vi "2 Round Buoy.vi"() -> ()   [LabVIEW 2011]
uses:
  2 Globals/2 Global.vi
  2 Typedefs/Velocity.ctl
  2 Typedefs/UTM Location.ctl
  2 Classes/Mission/Mission.lvclass
  2 Classes/MissionQueue/MissionQueue.lvclass
  2 Classes/Waypoint/Waypoint.lvclass
panel:
  in  "Tolerance":dbl=0.5
  out "First Waypoint":T1 {"North" format="%#_10f"; "East" format="%#_8f"}
  out "Third Waypoint":T1 {"North" format="%#_10f"; "East" format="%#_8f"}
  out "Second Waypoint":T1 {"North" format="%#_10f"; "East" format="%#_8f"}
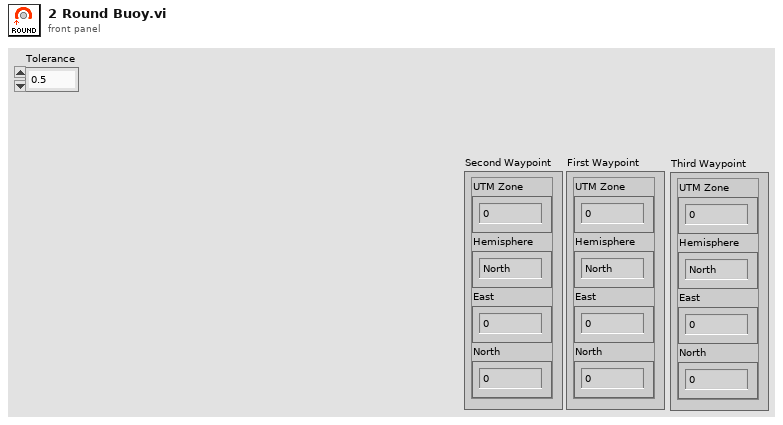
[diagram p1: front panel]
types:
  T1 = typedef "UTM Location.ctl" = cluster{"UTM Zone":dbl, "Hemisphere":enum16{"North", "South"}, "East":dbl, "North":dbl}
  T2 = typedef "Velocity.ctl" = cluster{"East":dbl, "North":dbl}
  T3 = cluster{"UTM Zone":dbl, "Hemisphere":u16, "East":dbl, "North":dbl}
  T4 = typedef "heading.ctl" = dbl
  T5 = typedef "Waypoints List.ctl" = refnum<class "Waypoint.lvclass">[]
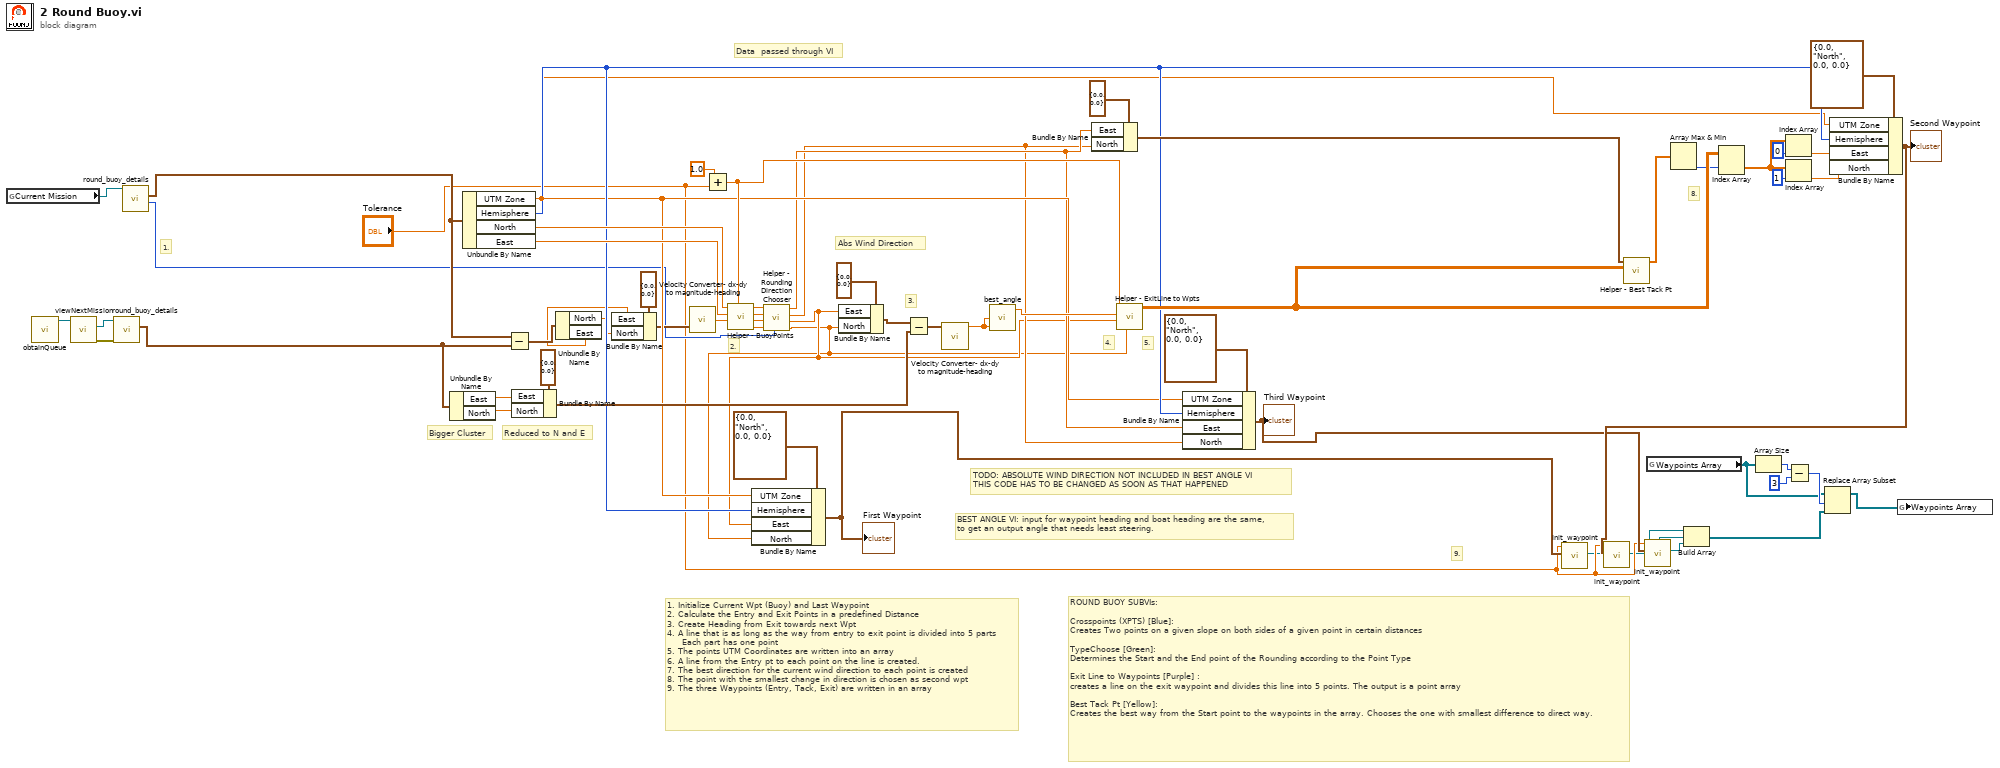
[diagram p0: block diagram]
diagram:
  # "ROUND BUOY SUBVIs:\n\nCrosspoints (XPTS) [Blue]:\nCreates Two points on a given slope on both sides of a given point in certain distances\n\nTypeChoose [Green]:\nDetermines the Start and the End point of the Rounding according to the Point Type\n\nExit Line to Waypoints [Purple] :\ncreates a line on the exit waypoint and divides this line into 5 points. The output is a point array\n\nBest Tack Pt [Yellow]:\nCreates the best way from the Start point to the waypoints in the array. Chooses the one with smallest difference to direct way."
  # "BEST ANGLE VI: input for waypoint heading and boat heading are the same,\nto get an output angle that needs least steering."
  # "Reduced to N and E"
  # "Bigger Cluster"
  # "Data  passed through VI"
  # "9."
  # "TODO: ABSOLUTE WIND DIRECTION NOT INCLUDED IN BEST ANGLE VI\nTHIS CODE HAS TO BE CHANGED AS SOON AS THAT HAPPENED"
  # "8."
  # "5."
  # "1. Initialize Current Wpt (Buoy) and Last Waypoint\n2. Calculate the Entry and Exit Points in a predefined Distance\n3. Create Heading from Exit towards next Wpt\n4. A line that is as long as the way from entry to exit point is divided into 5 parts\n     Each part has one point\n5. The points UTM Coordinates are written into an array\n6. A line from the Entry pt to each point on the line is created.\n7. The best direction for the current wind direction to each point is created\n8. The point with the smallest change in direction is chosen as second wpt\n9. The three Waypoints (Entry, Tack, Exit) are written in an array"
  # "4."
  # "3."
  # "Abs Wind Direction"
  # "2."
  # "1."
  n1 = global read "2 Global.vi" "Current Mission"() -> (w21:refnum<class "Mission.lvclass">)
  n2 = call "obtainQueue.vi"() -> ("MissionQueue.lvclass"=w15:refnum<class "MissionQueue.lvclass">)  [unwired: 10 in, 1 out]
  n3 = call "viewNextMission.vi"("MissionQueue in"=w15) -> ("error out"=w18:errorcluster, "Mission.lvclass"=w17:refnum<class "Mission.lvclass">)  [unwired: 7 in, 2 out]
  n4 = call-dynamic "round_buoy_details.vi"("error in (no error)"=w18, "Mission in"=w17) -> ("Buoy to Round"=w16:T1)  [unwired: 6 in, 3 out]
  n5 = call-dynamic "round_buoy_details.vi"("Mission in"=w21) -> ("Round side?"=w19:enum16{"Starboard", "Port"}, "Buoy to Round"=w20:T1)  [unwired: 7 in, 2 out]
  n6 = Unbundle By Name(w16) -> ("East"=w59:dbl, "North"=w58:dbl)
  n7 = Unbundle By Name(w20) -> ("UTM Zone"=w36:dbl, "Hemisphere"=w37:enum16{"North", "South"}, "North"=w62:dbl, "East"=w61:dbl)
  n8 = Subtract(x=w20, y=w16) -> (x-y=w26:T3)
  n9 = Bundle By Name(cluster=T2 {"East"=0.0, "North"=0.0} ("Vector In"), "East"=w59, "North"=w58) -> (w55:T2)
  n10 = Unbundle By Name(w26) -> ("North"=w24:dbl, "East"=w14:dbl)
  n11 = Bundle By Name(cluster=T2 {"East"=0.0, "North"=0.0} ("Vector In"), "East"=w14, "North"=w24) -> (w23:T2)
  n12 = call "Velocity Converter- dx-dy to magnitude-heading.vi"("Vector In"=w23) -> ("Heading Out"=w22:T4)  [unwired: 9 in, 1 out]
  n13 = Add(x=1.0, y="Tolerance") -> (x+y=w53:dbl)
  n14 = call "Helper - BuoyPoints.vi"("Distance"=w53, "K"=w22, "East"=w61, "North"=w62) -> ("NorthOut 2"=w31:dbl, "East Out 2"=w32:dbl, "NorthOut"=w33:dbl, "East Out"=w34:dbl)  [unwired: 4 in]
  n15 = call "Helper - Rounding Direction Chooser.vi"("Enum"=w19, "Point NORTH 2"=w31, "Point EAST 2"=w32, "Point NORTH"=w33, "Point EAST"=w34) -> ("End Point NORTH"=w27:dbl, "End Point EAST"=w28:dbl, "Start Point NORTH"=w29:dbl, "Start Point EAST"=w30:dbl)  [unwired: 3 in]
  n16 = Bundle By Name(cluster=T1 {"UTM Zone"=0.0, "Hemisphere"=enum."North", "East"=0.0, "North"=0.0} ("UTM Location"), "UTM Zone"=w36, "Hemisphere"=w37, "East"=w28, "North"=w27) -> (w13:T1)
  "First Waypoint" <- w13
  n17 = Bundle By Name(cluster=T2 {"East"=0.0, "North"=0.0} ("Vector In"), "East"=w28, "North"=w27) -> (w41:T2)
  n18 = Subtract(x=w41, y=w55) -> (x-y=w54:T2)
  n19 = call "Velocity Converter- dx-dy to magnitude-heading.vi"("Vector In"=w54) -> ("Heading Out"=w35:T4)  [unwired: 9 in, 1 out]
  n20 = call "best_angle.vi"("Waypoint Heading"=w35, "Current Heading"=w35) -> ("Best Angle"=w52:dbl)  [unwired: 1 in, 2 out]
  n21 = Bundle By Name(cluster=T2 {"East"=0.0, "North"=0.0} ("Vector In"), "East"=w30, "North"=w29) -> (w42:T2)
  n22 = call "Helper - ExitLine to Wpts.vi"("NorthOut in"=w27, "East Out in"=w28, "Best Angle"=w52, "Dist/Time"=w53) -> ("Point on Line"=w49:dbl[][])  [unwired: 7 in]
  n23 = Bundle By Name(cluster=T1 {"UTM Zone"=0.0, "Hemisphere"=enum."North", "East"=0.0, "North"=0.0} ("UTM Location"), "UTM Zone"=w36, "Hemisphere"=w37, "East"=w30, "North"=w29) -> (w11:T1)
  "Third Waypoint" <- w11
  n24 = call "init_waypoint.vi"("Coords"=w13, "Tolerance (m)"="Tolerance") -> ("Waypoint Out"=w8:refnum<class "Waypoint.lvclass">)  [unwired: 9 in]
  n25 = call "Helper - Best Tack Pt.vi"("Point on Line"=w49, "Vector In"=w42) -> ("Array"=w50:dbl[])  [unwired: 9 in]
  n26 = call "init_waypoint.vi"("Coords"=w11, "Tolerance (m)"="Tolerance") -> ("Waypoint Out"=w6:refnum<class "Waypoint.lvclass">)  [unwired: 9 in]
  n27 = global read "2 Global.vi" "Waypoints Array"() -> (w3:T5)
  n28 = Array Max & Min(array=w50) -> (min index (indices)=w48:i32)  [unwired: 3 out]
  n29 = Index Array(array=w49, index (row)=w48) -> (element=w43:dbl[])  [unwired: 1 in]
  n30 = Array Size(array=w3) -> (size(s)=w9:i32)
  n31 = Index Array(array=w43, index=0) -> (element=w45:dbl)
  n32 = Index Array(array=w43, index=1) -> (element=w44:dbl)
  n33 = Subtract(x=w9, y=3) -> (x-y=w4:i32)
  n34 = Bundle By Name(cluster=T1 {"UTM Zone"=0.0, "Hemisphere"=enum."North", "East"=0.0, "North"=0.0} ("UTM Location"), "UTM Zone"=w36, "Hemisphere"=w37, "East"=w45, "North"=w44) -> (w12:T1)
  "Second Waypoint" <- w12
  n35 = call "init_waypoint.vi"("Coords"=w12, "Tolerance (m)"="Tolerance") -> ("Waypoint Out"=w7:refnum<class "Waypoint.lvclass">)  [unwired: 9 in]
  n36 = Build Array(w8, w7, w6) -> (w2:refnum<class "Waypoint.lvclass">[])
  n37 = Replace Array Subset(array=w3, new element=w2, index=w4) -> (w1:T5)
  n38 = global write "2 Global.vi" "Waypoints Array"(w1) -> ()
